vi "CountPulses10.vi"(10 "10bit input":bool[](array[boolean])=[FALSE, FALSE, FALSE, FALSE, FALSE, FALSE, FALSE, FALSE, FALSE, FALSE], 11 "Last sample":bool) -> (2 "No. of detected pulses":u16, 3 "New last sample":bool)   [LabVIEW 2012]
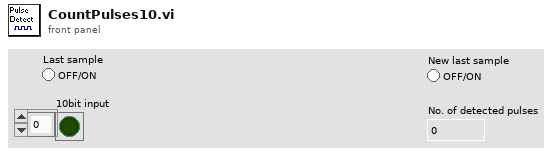
[diagram p1: front panel]
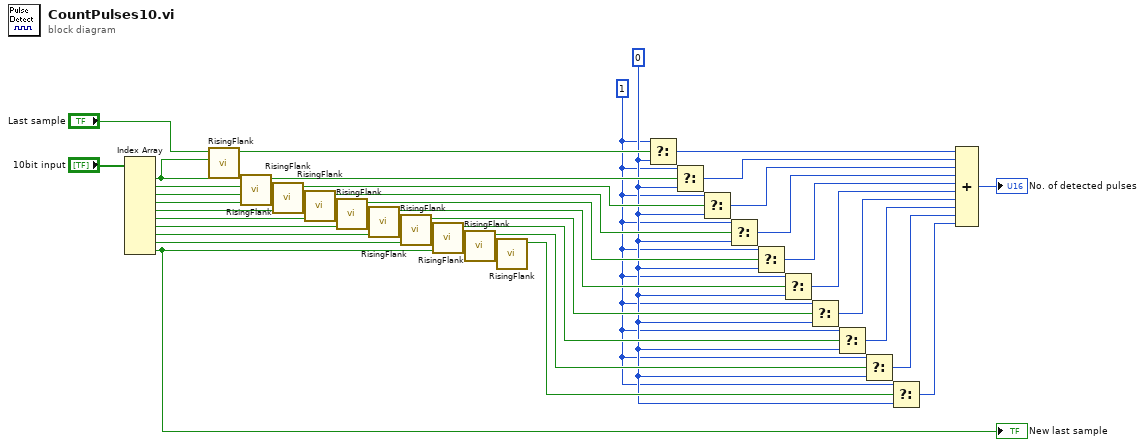
[diagram p0: block diagram]
diagram:
  w14 = u16 1
  w15 = u16 0
  n1 = Index Array(array="10bit input") -> (element #1=w1:bool, element #2=w34:bool, element #3=w33:bool, element #4=w32:bool, element #5=w31:bool, element #6=w30:bool, element #7=w29:bool, element #8=w28:bool, element #9=w27:bool, element #10=w26:bool)  [unwired: 10 in]
  "New last sample" <- w26
  n2 = call "RisingFlank.vi"("2nd sample"=w1, "1st sample"="Last sample") -> ("Rising flank?"=w25:bool)  [unwired: 7 in]
  n3 = call "RisingFlank.vi"("2nd sample"=w34, "1st sample"=w1) -> ("Rising flank?"=w24:bool)  [unwired: 7 in]
  n4 = call "RisingFlank.vi"("2nd sample"=w33, "1st sample"=w34) -> ("Rising flank?"=w23:bool)  [unwired: 7 in]
  n5 = call "RisingFlank.vi"("2nd sample"=w32, "1st sample"=w33) -> ("Rising flank?"=w22:bool)  [unwired: 7 in]
  n6 = call "RisingFlank.vi"("2nd sample"=w31, "1st sample"=w32) -> ("Rising flank?"=w21:bool)  [unwired: 7 in]
  n7 = call "RisingFlank.vi"("2nd sample"=w30, "1st sample"=w31) -> ("Rising flank?"=w20:bool)  [unwired: 7 in]
  n8 = call "RisingFlank.vi"("2nd sample"=w29, "1st sample"=w30) -> ("Rising flank?"=w19:bool)  [unwired: 7 in]
  n9 = call "RisingFlank.vi"("2nd sample"=w28, "1st sample"=w29) -> ("Rising flank?"=w18:bool)  [unwired: 7 in]
  n10 = call "RisingFlank.vi"("2nd sample"=w27, "1st sample"=w28) -> ("Rising flank?"=w17:bool)  [unwired: 7 in]
  n11 = call "RisingFlank.vi"("2nd sample"=w26, "1st sample"=w27) -> ("Rising flank?"=w16:bool)  [unwired: 7 in]
  n12 = Select(t=w14, s=w25, f=w15) -> (s? t:f=w13:u16)
  n13 = Select(t=w14, s=w24, f=w15) -> (s? t:f=w12:u16)
  n14 = Select(t=w14, s=w23, f=w15) -> (s? t:f=w11:u16)
  n15 = Select(t=w14, s=w22, f=w15) -> (s? t:f=w10:u16)
  n16 = Select(t=w14, s=w21, f=w15) -> (s? t:f=w9:u16)
  n17 = Select(t=w14, s=w20, f=w15) -> (s? t:f=w8:u16)
  n18 = Select(t=w14, s=w19, f=w15) -> (s? t:f=w7:u16)
  n19 = Select(t=w14, s=w18, f=w15) -> (s? t:f=w6:u16)
  n20 = Select(t=w14, s=w17, f=w15) -> (s? t:f=w5:u16)
  n21 = Select(t=w14, s=w16, f=w15) -> (s? t:f=w4:u16)
  n22 = Compound Arithmetic op=ADD(w13, w12, w11, w10, w9, w8, w7, w6, w5, w4) -> (→"No. of detected pulses":u16)
